vi "Read Packet.vi"(8 "error in (no error)":errorcluster, 10 "capture_data":string, 11 "pcap reference":u32) -> (0 "error out":errorcluster, 1 "timed out":bool, 2 "capture_data out":string, 3 "pcap reference out":u32, 4 "capture_len":u32, 6 "timestamp":cluster{"tv_sec":u32, "tv_usec":u32})   [LabVIEW 2017, in "lvwpcap.lvlib"]
doc: "This VI reads an ethernet packet. It outputs the packet in the form of a raw string."
uses:
  lvwpcap.lvlib
  LVpcap.dll
panel:
  out "return type":i32
  in  "capture_len (dummy)":u32
  in  "tv_usec (dummy)":u32
  in  "tv_sec (dummy)":u32
  # "Select Help»Show Context Help and move the cursor over the VI icon to display help for this VI."
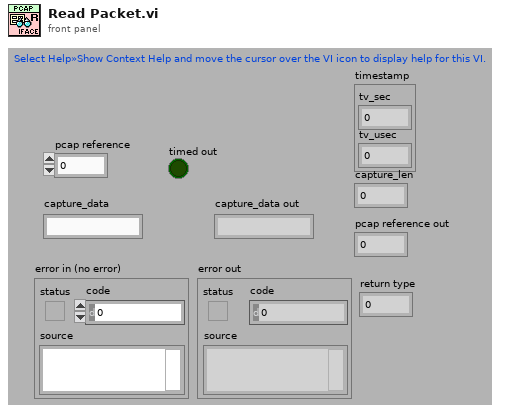
[diagram p1: front panel]
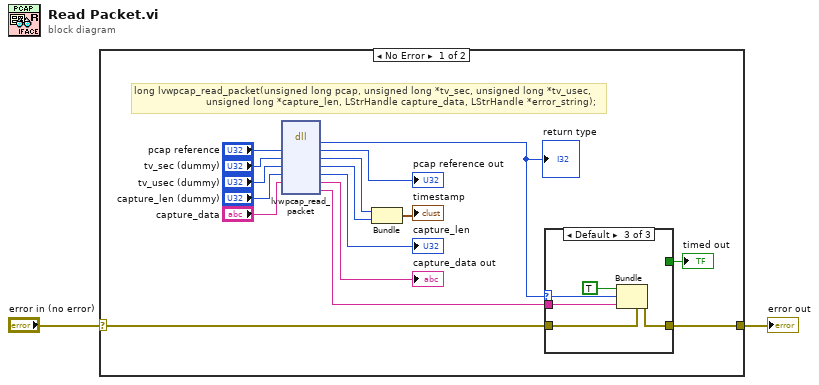
[diagram p0: block diagram]
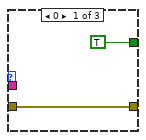
[diagram p2: hidden frame]
diagram:
  n1 = case shown="No Error" "error in (no error)" {
    selector: "error in (no error)" -> [w3 w27]
    tunnel: [w18 w27] -> w2
    frame No Error {
      # "long lvwpcap_read_packet(unsigned long pcap, unsigned long *tv_sec, unsigned long *tv_usec,\n                        unsigned long *capture_len, LStrHandle capture_data, LStrHandle *error_string);"
      n2 = dll-call lib="C:/Users/Michaello/Desktop/MGR NOWEEEEEEEEEEEEEE/MR PROFINET 2017/Lib/WinPcap/LVpcap.dll" fn="lvwpcap_read_packet"("pcap"="pcap reference", "tv_sec"="tv_sec (dummy)", "tv_usec"="tv_usec (dummy)", "capture_len"="capture_len (dummy)", "capture_data"="capture_data") -> ("return type"=w17:i32, "pcap"=→"pcap reference out":u32, "tv_sec"=w11:u32, "tv_usec"=w10:u32, "capture_len"=→"capture_len":u32, "capture_data"=→"capture_data out":string, "error_string"=w5:string)  [unwired: 4 in, 2 out]
      "return type" <- w17
      n3 = Bundle("tv_sec"=w11, "tv_usec"=w10) -> (→"timestamp":cluster{"tv_sec":u32, "tv_usec":u32})  [unwired: 1 in]
      n4 = case shown="Default" w17 {
        selector: w17 -> [_ _ w25]
        tunnel: w5 -> [_ _ w24]
        tunnel: w3 -> [w20 w21 w26]
        tunnel: [w20 w21 w22] -> w18
        tunnel: [TRUE _ _] -> w7
        frame 0 {
        }
        frame 1 {
        }
        frame Default {
          n5 = Bundle(cluster=w26, "status"=TRUE, "code"=w25, "source"=w24) -> (w22:errorcluster)
        }
      }
      "timed out" <- w7
    }
    frame Error {
    }
  }
  "error out" <- w2
